vi "Offset.vi"(8 "error in (no error)":errorcluster, 9 "y offset":dbl, 10 "x offset":dbl, 11 "Multiple XY-data in":cluster{"X-array":dbl[], "Y-array":dbl[]}[](array[cluster]) {"Y-array" format="%.2p"; "X-array" format="%.2p"}) -> (0 "error out":errorcluster, 3 "Multiple XY-data out":cluster{"X-array":dbl[], "Y-array":dbl[]}[](array[cluster]) {"Y-array" format="%.2p"; "X-array" format="%.2p"})   [LabVIEW 2016, in "xy_utilities.lvlib"]
uses:
  xy_utilities.lvlib
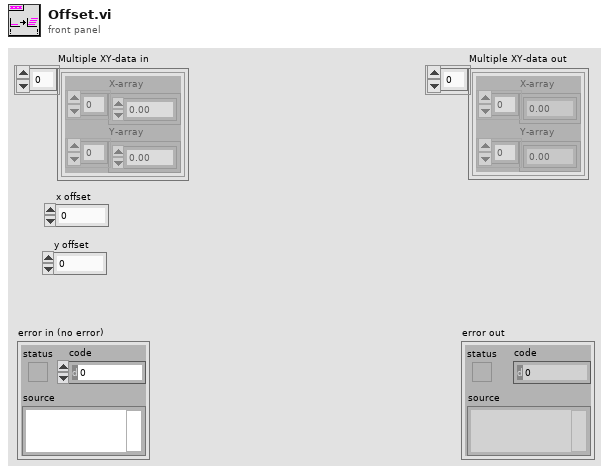
[diagram p1: front panel]
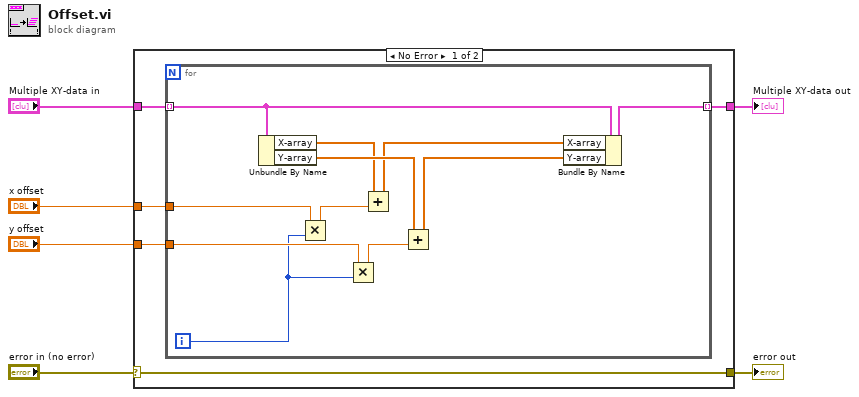
[diagram p0: block diagram]
diagram:
  n1 = case shown="No Error" "error in (no error)" {
    selector: "error in (no error)" -> [w11 w24]
    tunnel: [w11 w24] -> w5
    tunnel: "Multiple XY-data in" -> [w10 w23]
    tunnel: [w9 w23] -> w3
    tunnel: "y offset" -> [w8 _]
    tunnel: "x offset" -> [w7 _]
    frame No Error {
      n2 = for {
        tunnel: w10 -> [w22] mode=indexing
        tunnel: [w21] -> w9 mode=indexing
        tunnel: w8 -> [w18]
        tunnel: w7 -> [w14]
        i -> [w16]
        n3 = Unbundle By Name(w22) -> ("X-array"=w13:dbl[], "Y-array"=w20:dbl[])
        n4 = Multiply(x=w14, y=w16) -> (x*y=w15:dbl)
        n5 = Multiply(x=w18, y=w16) -> (x*y=w17:dbl)
        n6 = Add(x=w13, y=w15) -> (x+y=w12:dbl[])
        n7 = Add(x=w20, y=w17) -> (x+y=w19:dbl[])
        n8 = Bundle By Name(cluster=w22, "X-array"=w12, "Y-array"=w19) -> (w21:cluster{"X-array":dbl[], "Y-array":dbl[]})
      }
    }
    frame Error {
    }
  }
  "error out" <- w5
  "Multiple XY-data out" <- w3
